vi "VI Tree.vi"   [LabVIEW 2021, in "Field_RnD_Services_LIBSSH2_Toolkit.lvlib"]
doc: "Shows all of the public VIs for the toolkit grouped by LabVIEW class in the block diagram."
uses:
  Field_RnD_Services_LIBSSH2_Toolkit.lvlib
  SSH/SSH.lvclass
  Agent Identity/Agent Identity.lvclass
  Agent/Agent.lvclass
  Channel/Channel.lvclass
  File Info/File Info.lvclass
  Known Host/Known Host.lvclass
  Channel/Support/Destroy to Listener.vi
  File Info/Support/Create from Session.vi
  Channel/Support/Create from Listener.vi
  Agent Identity/Support/Create from Agent.vi
  Agent/Support/Create from Session.vi
  Agent/Support/Destroy to Session.vi
  Agent Identity/Support/Destroy to Agent.vi
  Known Hosts/Known Hosts.lvclass
  Listener/Listener.lvclass
  Session/Session.lvclass
  SFTP Attributes/SFTP Attributes.lvclass
  SFTP Directory/SFTP Directory.lvclass
  SFTP File/SFTP File.lvclass
  SFTP/SFTP.lvclass
  Session/Support/Create from SSH.vi
  Session/Support/Password Authentication.vi
  Session/Support/Destroy to SSH.vi
  Known Hosts/Support/Create from Session.vi
  Known Host/Support/Destroy to Known Hosts.vi
  Known Host/Support/Create from Known Hosts.vi
  Known Hosts/Support/Destroy to Session.vi
  Listener/Support/Destroy to Session.vi
  Listener/Support/Create from Session.vi
  SFTP File/Support/Close to SFTP.vi
  SFTP Directory/Support/Open from SFTP.vi
  SFTP File/Support/Open from SFTP.vi
  SFTP/Support/Create from Session.vi
  SFTP/Support/Destroy to Session.vi
  SFTP/Support/Resolve Symbolic Link.vi
  SFTP Directory/Support/Close to SFTP.vi
  SFTP Attributes/Support/Destroy to SFTP Directory.vi
  SFTP Attributes/Support/Create from SFTP Directory.vi
  File Info/Support/Destroy to Session.vi
panel:
  # "Copyright (c) 2019 Field R&D Services, LLC\n\nLicensed under the Apache License, Version 2.0 (the \"License\"); you may not use this file except in compliance with the License.  You may obtain a copy of the License at\n\nhttp://www.apache.org/licenses/LICENSE-2.0\n\nUnless required by applicable law or agreed to in writing, software distributed under the License is distributed on an \"AS IS\" BASIS, WITHOUT WARRANTIES OR CONDITIONS OF ANY KIND, either express or implied.  See the License for the specific language governing permissions and limitations under the License.\n\nLIBSSH2-LabVIEW is licensed under either the BSD-3-Clause (https://opensource.org/licenses/BSD-3-Clause) or the Apache-2.0 license, http://www.apache.org/licenses/LICENSE-2.0, and it contains statically compiled code from the libssh2 (https://github.com/libssh2/libssh2) and OpenSSL (https://github.com/openssl/openssl) projects, which are licensed under the MIT license (https://github.com/libssh2/libssh2/blob/master/COPYING) and the Apache-2.0 license, https://github.com/openssl/openssl/blob/master/LICENSE, respectively."
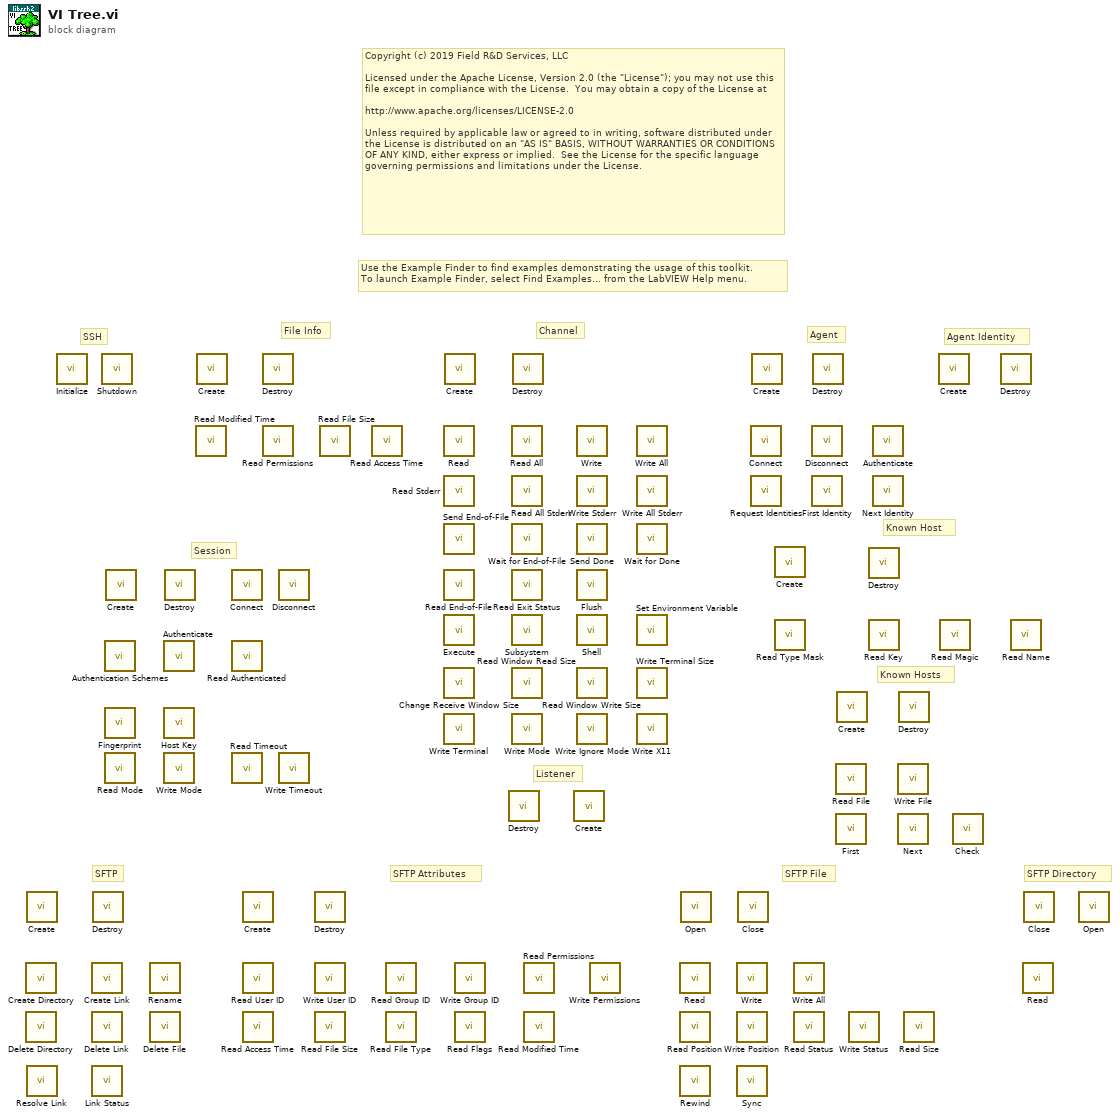
[diagram p0: block diagram]
diagram:
  # "SFTP"
  # "SFTP File"
  # "SFTP Directory"
  # "SFTP Attributes"
  # "Use the Example Finder to find examples demonstrating the usage of this toolkit.\nTo launch Example Finder, select Find Examples... from the LabVIEW Help menu."
  # "Session"
  # "Listener"
  # "Known Hosts"
  # "Known Host"
  # "File Info"
  # "Channel"
  # "Agent"
  # "Agent Identity"
  # "SSH"
  # "Copyright (c) 2019 Field R&D Services, LLC\n\nLicensed under the Apache License, Version 2.0 (the \"License\"); you may not use this file except in compliance with the License.  You may obtain a copy of the License at\n\nhttp://www.apache.org/licenses/LICENSE-2.0\n\nUnless required by applicable law or agreed to in writing, software distributed under the License is distributed on an \"AS IS\" BASIS, WITHOUT WARRANTIES OR CONDITIONS OF ANY KIND, either express or implied.  See the License for the specific language governing permissions and limitations under the License."
  n1 = call "Create Directory.vi"() -> ()  [unwired: 10 in, 2 out]
  n2 = call "Delete Directory.vi"() -> ()  [unwired: 10 in, 2 out]
  n3 = call-poly "Create.vi"() -> ()  [unwired: 10 in, 2 out]
  n4 = call-poly "Resolve Link.vi"() -> ()  [unwired: 9 in, 3 out]
  n5 = call "Initialize.vi"() -> ()  [unwired: 10 in, 2 out]
  n6 = call "Create Link.vi"() -> ()  [unwired: 10 in, 2 out]
  n7 = call "Delete Link.vi"() -> ()  [unwired: 10 in, 2 out]
  n8 = call "Link Status.vi"() -> ()  [unwired: 9 in, 3 out]
  n9 = call-poly "Destroy.vi"() -> ()  [unwired: 10 in, 2 out]
  n10 = call "Shutdown.vi"() -> ()  [unwired: 11 in, 1 out]
  n11 = call "Authentication Schemes.vi"() -> ()  [unwired: 9 in, 3 out]
  n12 = call "Fingerprint.vi"() -> ()  [unwired: 9 in, 3 out]
  n13 = call "Read Mode.vi"() -> ()  [unwired: 9 in, 3 out]
  n14 = call-poly "Create.vi"() -> ()  [unwired: 10 in, 2 out]
  n15 = call "Rename.vi"() -> ()  [unwired: 10 in, 2 out]
  n16 = call "Delete File.vi"() -> ()  [unwired: 10 in, 2 out]
  n17 = call-poly "Authenticate.vi"() -> ()  [unwired: 10 in, 2 out]
  n18 = call "Host Key.vi"() -> ()  [unwired: 8 in, 4 out]
  n19 = call "Write Mode.vi"() -> ()  [unwired: 10 in, 2 out]
  n20 = call-poly "Destroy.vi"() -> ()  [unwired: 10 in, 2 out]
  n21 = call "Read Modified Time.vi"() -> ()  [unwired: 9 in, 3 out]
  n22 = call-poly "Create.vi"() -> ()  [unwired: 9 in, 3 out]
  n23 = call "Connect.vi"() -> ()  [unwired: 10 in, 2 out]
  n24 = call "Read Authenticated.vi"() -> ()  [unwired: 9 in, 3 out]
  n25 = call "Read Timeout.vi"() -> ()  [unwired: 9 in, 3 out]
  n26 = call-poly "Create.vi"() -> ()  [unwired: 9 in, 3 out]
  n27 = call "Read User ID.vi"() -> ()  [unwired: 9 in, 3 out]
  n28 = call "Read Access Time.vi"() -> ()  [unwired: 9 in, 3 out]
  n29 = call-poly "Destroy.vi"() -> ()  [unwired: 10 in, 2 out]
  n30 = call "Read Permissions.vi"() -> ()  [unwired: 9 in, 3 out]
  n31 = call "Disconnect.vi"() -> ()  [unwired: 10 in, 2 out]
  n32 = call "Write Timeout.vi"() -> ()  [unwired: 10 in, 2 out]
  n33 = call-poly "Destroy.vi"() -> ()  [unwired: 10 in, 2 out]
  n34 = call "Write User ID.vi"() -> ()  [unwired: 10 in, 2 out]
  n35 = call "Read File Size.vi"() -> ()  [unwired: 9 in, 3 out]
  n36 = call "Read File Size.vi"() -> ()  [unwired: 9 in, 3 out]
  n37 = call "Read Access Time.vi"() -> ()  [unwired: 9 in, 3 out]
  n38 = call "Read Group ID.vi"() -> ()  [unwired: 9 in, 3 out]
  n39 = call "Read File Type.vi"() -> ()  [unwired: 9 in, 3 out]
  n40 = call "Read.vi"() -> ()  [unwired: 9 in, 3 out]
  n41 = call "Read Stderr.vi"() -> ()  [unwired: 9 in, 3 out]
  n42 = call "Send End-of-File.vi"() -> ()  [unwired: 10 in, 2 out]
  n43 = call "Read End-of-File.vi"() -> ()  [unwired: 9 in, 3 out]
  n44 = call "Execute.vi"() -> ()  [unwired: 10 in, 2 out]
  n45 = call "Change Receive Window Size.vi"() -> ()  [unwired: 9 in, 3 out]
  n46 = call "Write Terminal.vi"() -> ()  [unwired: 10 in, 2 out]
  n47 = call-poly "Create.vi"() -> ()  [unwired: 10 in, 2 out]
  n48 = call "Write Group ID.vi"() -> ()  [unwired: 10 in, 2 out]
  n49 = call "Read Flags.vi"() -> ()  [unwired: 9 in, 3 out]
  n50 = call-poly "Destroy.vi"() -> ()  [unwired: 10 in, 2 out]
  n51 = call "Read All.vi"() -> ()  [unwired: 8 in, 4 out]
  n52 = call "Read All Stderr.vi"() -> ()  [unwired: 8 in, 4 out]
  n53 = call "Wait for End-of-File.vi"() -> ()  [unwired: 10 in, 2 out]
  n54 = call "Read Exit Status.vi"() -> ()  [unwired: 9 in, 3 out]
  n55 = call "Subsystem.vi"() -> ()  [unwired: 10 in, 2 out]
  n56 = call "Read Window Read Size.vi"() -> ()  [unwired: 9 in, 3 out]
  n57 = call "Write Mode.vi"() -> ()  [unwired: 10 in, 2 out]
  n58 = call-poly "Destroy.vi"() -> ()  [unwired: 10 in, 2 out]
  n59 = call "Read Permissions.vi"() -> ()  [unwired: 9 in, 3 out]
  n60 = call "Read Modified Time.vi"() -> ()  [unwired: 9 in, 3 out]
  n61 = call-poly "Create.vi"() -> ()  [unwired: 10 in, 2 out]
  n62 = call "Write.vi"() -> ()  [unwired: 9 in, 3 out]
  n63 = call "Write Stderr.vi"() -> ()  [unwired: 9 in, 3 out]
  n64 = call "Send Done.vi"() -> ()  [unwired: 10 in, 2 out]
  n65 = call "Flush.vi"() -> ()  [unwired: 10 in, 2 out]
  n66 = call "Shell.vi"() -> ()  [unwired: 10 in, 2 out]
  n67 = call "Read Window Write Size.vi"() -> ()  [unwired: 9 in, 3 out]
  n68 = call "Write Ignore Mode.vi"() -> ()  [unwired: 10 in, 2 out]
  n69 = call "Write Permissions.vi"() -> ()  [unwired: 10 in, 2 out]
  n70 = call "Write All.vi"() -> ()  [unwired: 8 in, 4 out]
  n71 = call "Write All Stderr.vi"() -> ()  [unwired: 8 in, 4 out]
  n72 = call "Wait for Done.vi"() -> ()  [unwired: 10 in, 2 out]
  n73 = call "Set Environment Variable.vi"() -> ()  [unwired: 10 in, 2 out]
  n74 = call "Write Terminal Size.vi"() -> ()  [unwired: 10 in, 2 out]
  n75 = call "Write X11.vi"() -> ()  [unwired: 10 in, 2 out]
  n76 = call "Read.vi"() -> ()  [unwired: 9 in, 3 out]
  n77 = call "Read Position.vi"() -> ()  [unwired: 9 in, 3 out]
  n78 = call "Rewind.vi"() -> ()  [unwired: 10 in, 2 out]
  n79 = call-poly "Open.vi"() -> ()  [unwired: 10 in, 2 out]
  n80 = call "Write.vi"() -> ()  [unwired: 9 in, 3 out]
  n81 = call "Write Position.vi"() -> ()  [unwired: 10 in, 2 out]
  n82 = call "Sync.vi"() -> ()  [unwired: 10 in, 2 out]
  n83 = call-poly "Close.vi"() -> ()  [unwired: 9 in, 3 out]
  n84 = call "Connect.vi"() -> ()  [unwired: 10 in, 2 out]
  n85 = call "Request Identities.vi"() -> ()  [unwired: 10 in, 2 out]
  n86 = call-poly "Create.vi"() -> ()  [unwired: 10 in, 2 out]
  n87 = call-poly "Create.vi"() -> ()  [unwired: 9 in, 3 out]
  n88 = call "Read Type Mask.vi"() -> ()  [unwired: 9 in, 3 out]
  n89 = call "Write All.vi"() -> ()  [unwired: 9 in, 3 out]
  n90 = call "Read Status.vi"() -> ()  [unwired: 9 in, 3 out]
  n91 = call "Disconnect.vi"() -> ()  [unwired: 10 in, 2 out]
  n92 = call "First Identity.vi"() -> ()  [unwired: 8 in, 4 out]
  n93 = call-poly "Destroy.vi"() -> ()  [unwired: 10 in, 2 out]
  n94 = call "Read File.vi"() -> ()  [unwired: 9 in, 3 out]
  n95 = call "First.vi"() -> ()  [unwired: 8 in, 4 out]
  n96 = call-poly "Create.vi"() -> ()  [unwired: 10 in, 2 out]
  n97 = call "Write Status.vi"() -> ()  [unwired: 9 in, 3 out]
  n98 = call-poly "Destroy.vi"() -> ()  [unwired: 10 in, 2 out]
  n99 = call "Read Key.vi"() -> ()  [unwired: 9 in, 3 out]
  n100 = call "Authenticate.vi"() -> ()  [unwired: 9 in, 3 out]
  n101 = call "Next Identity.vi"() -> ()  [unwired: 7 in, 5 out]
  n102 = call "Write File.vi"() -> ()  [unwired: 10 in, 2 out]
  n103 = call "Next.vi"() -> ()  [unwired: 7 in, 5 out]
  n104 = call-poly "Destroy.vi"() -> ()  [unwired: 10 in, 2 out]
  n105 = call "Read Size.vi"() -> ()  [unwired: 9 in, 3 out]
  n106 = call-poly "Create.vi"() -> ()  [unwired: 9 in, 3 out]
  n107 = call "Read Magic.vi"() -> ()  [unwired: 9 in, 3 out]
  n108 = call "Check.vi"() -> ()  [unwired: 9 in, 3 out]
  n109 = call-poly "Destroy.vi"() -> ()  [unwired: 10 in, 2 out]
  n110 = call "Read Name.vi"() -> ()  [unwired: 9 in, 3 out]
  n111 = call "Read.vi"() -> ()  [unwired: 7 in, 5 out]
  n112 = call-poly "Close.vi"() -> ()  [unwired: 9 in, 3 out]
  n113 = call-poly "Open.vi"() -> ()  [unwired: 10 in, 2 out]
